vi "Define Queues and Events.vi"(8 "Error In":errorcluster, 9 "Max no of Traces in Queue":i32=1000, 10 "Initialization States":T1[](array[typedef])) -> (0 "Eror Out":errorcluster, 1 "Next State Queue":refnum<queue>, 3 "User Events":refnum<user-event>)   [LabVIEW 2017]
uses:
  Controls/DAQ States.ctl
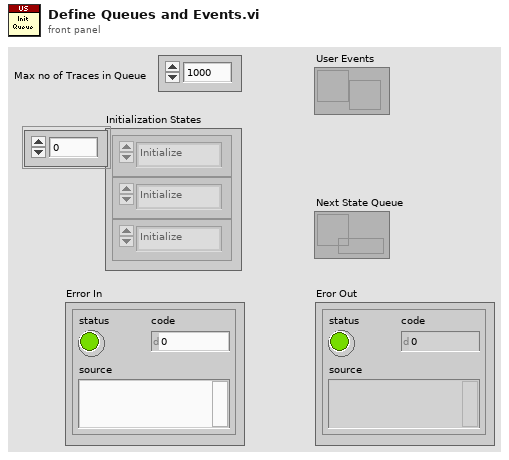
[diagram p1: front panel]
types:
  T1 = typedef "DAQ States.ctl" = enum16{"Initialize", "Idle", "Set Horizontal", "Set Vertical", "Set Trigger", "Set Display", "Acquire", "Analyze", "Set Switch", "Shutdown", "Quit"}
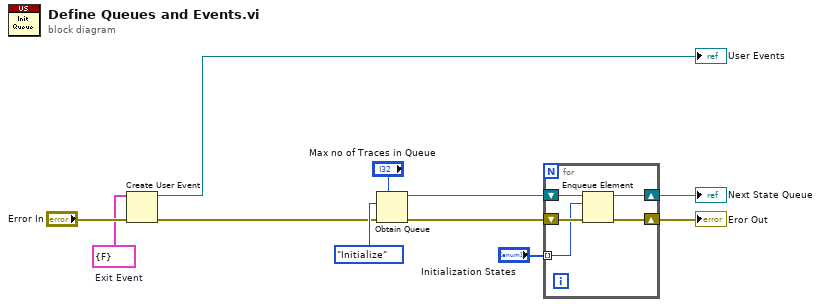
[diagram p0: block diagram]
diagram:
  w3 = cluster{"Exit":bool} {"Exit"=FALSE}  # Exit Event
  n1 = Create User Event(user event datatype=w3, error in="Error In") -> (user event=→"User Events":refnum<user-event>, error out=w1:errorcluster)
  n2 = Obtain Queue(max queue size (-1, unlimited)="Max no of Traces in Queue", element data type=DAQ_States."Initialize", error in (no error)=w1) -> (queue out=w6:refnum<queue>, error out=w2:errorcluster)  [unwired: 2 in, 1 out]
  n3 = for {
    shift-right: [w14] -> w8
    shift-left: w2 -> [w16]
    shift-right: [w15] -> w5
    shift-left: w6 -> [w13]
    tunnel: "Initialization States" -> [w12] mode=indexing
    n4 = Enqueue Element(queue=w13, element=w12, error in (no error)=w16) -> (queue out=w15:refnum<queue>, error out=w14:errorcluster)  [unwired: 1 in, 1 out]
  }
  "Eror Out" <- w8
  "Next State Queue" <- w5
